vi "FlywheelVariableAngleControl.vi"(10 "Flywheel Commands":T1, 11 "Inputs_FlyWheel":T2={"Speed"=0.0, "Target Distance"=142.3980439543401}) -> (3 "Outputs_Flywheel":T3={"Wheel Speed"=9001.0})   [LabVIEW 2012]
uses:
  Outputs_Flywheel.ctl
  Sensor_Inputs_FlyWheel.ctl
  Input_Commands_Flywheel.ctl
panel:
  in  "Key Speed":dbl=2550.0
  in  "Reverse Speed":dbl=-400.0
  in  "Reset Speed":dbl=1300.0
  in  "Layup Speed":dbl=1300.0
  out "D out":dbl
  out "I out":dbl=0.003692626953125
  out "P out":dbl=0.399993896484375
  in  "Get PID":bool
  out "error out 2":errorcluster
  out "error out":errorcluster
  out "Average Speed":dbl
  in  "D":dbl
  in  "I":dbl=0.0037
  in  "P":dbl=0.6
  in  "SetPID":bool
  in  "Wheel Speed":dbl
  out "Current Speed":dbl(graph)
  # "Inputs"
  # "Constants"
  # "Outputs"
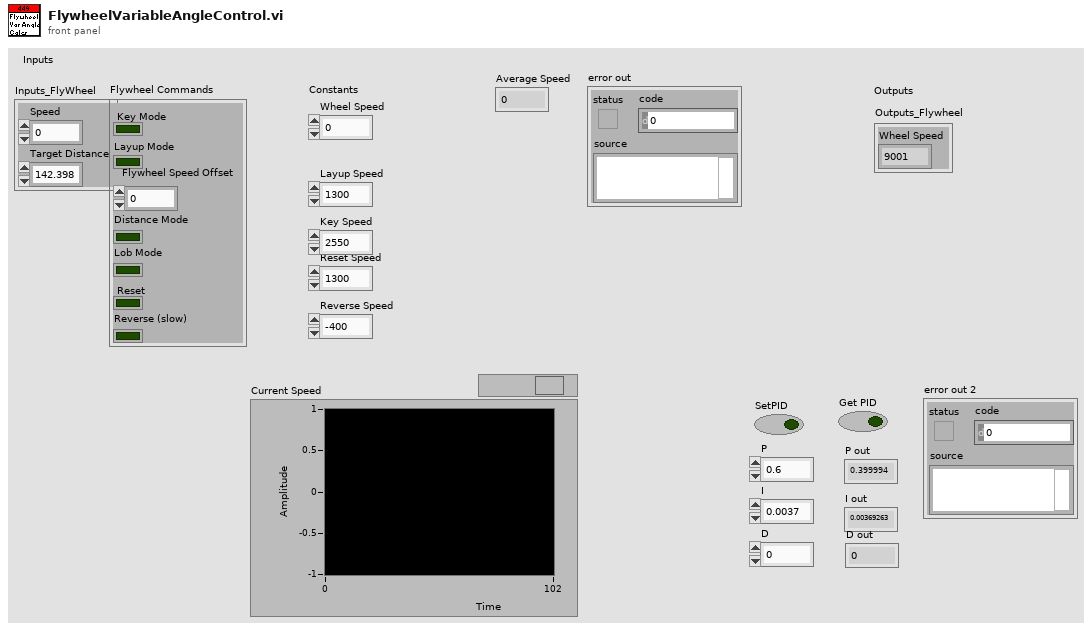
[diagram p1: front panel]
types:
  T1 = typedef "Input_Commands_Flywheel.ctl" = cluster{"Key Mode":bool, "Layup Mode":bool, "Flywheel Speed Offset":dbl, "Distance Mode":bool, "Lob Mode":bool, "Reset":bool, "Reverse (slow)":bool}
  T2 = typedef "Sensor_Inputs_FlyWheel.ctl" = cluster{"Speed":dbl, "Target Distance":dbl}
  T3 = typedef "Outputs_Flywheel.ctl" = cluster{"Wheel Speed":dbl}
  T4 = typedef "WPI_MotorControlDeviceRef.ctl" = cluster{"DeviceStatus":errorcluster, "Type":enum16{"PWM", "CAN"}, "PWM":cluster{"Digital Module":T5, "PWM Channel":T6, "DeadBand":T7}, "CAN":cluster{"Device Number":u8, "Control Mode":T8, "Semaphore":T9, "Max Vout":dbl}, "Invert":bool, "TransformRef":T10, "InvTransformRef":T10}
  T5 = typedef "FPGA_TypedefDigitalModule.ctl" = enum16{"Digital Module 1", "Digital Module 2"}
  T6 = typedef "FPGA_DIOPWMChannel.ctl" = enum8{"PWM 1", "PWM 2", "PWM 3", "PWM 4", "PWM 5", "PWM 6", "PWM 7", "PWM 8", "PWM 9", "PWM 10", "Invalid"}
  T7 = typedef "WPI_PWMDeadband.ctl" = cluster{"Name":string, "maxPositivePwm":i32, "minPositivePwm":i32, "centerPwm":i32, "maxNegativePwm":i32, "minNegativePwm":i32, "angularRange":u16}
  T8 = typedef "WPI_CANJaguar_ControlMode.ctl" = enum8{"Percent VBus", "Current", "Speed", "Position", "Voltage"}
  T9 = typedef "Semaphore RefNum" = refnum<k1>
  T10 = typedef "WPI_PWMTransform_ConPane.ctl" = refnum<vi>
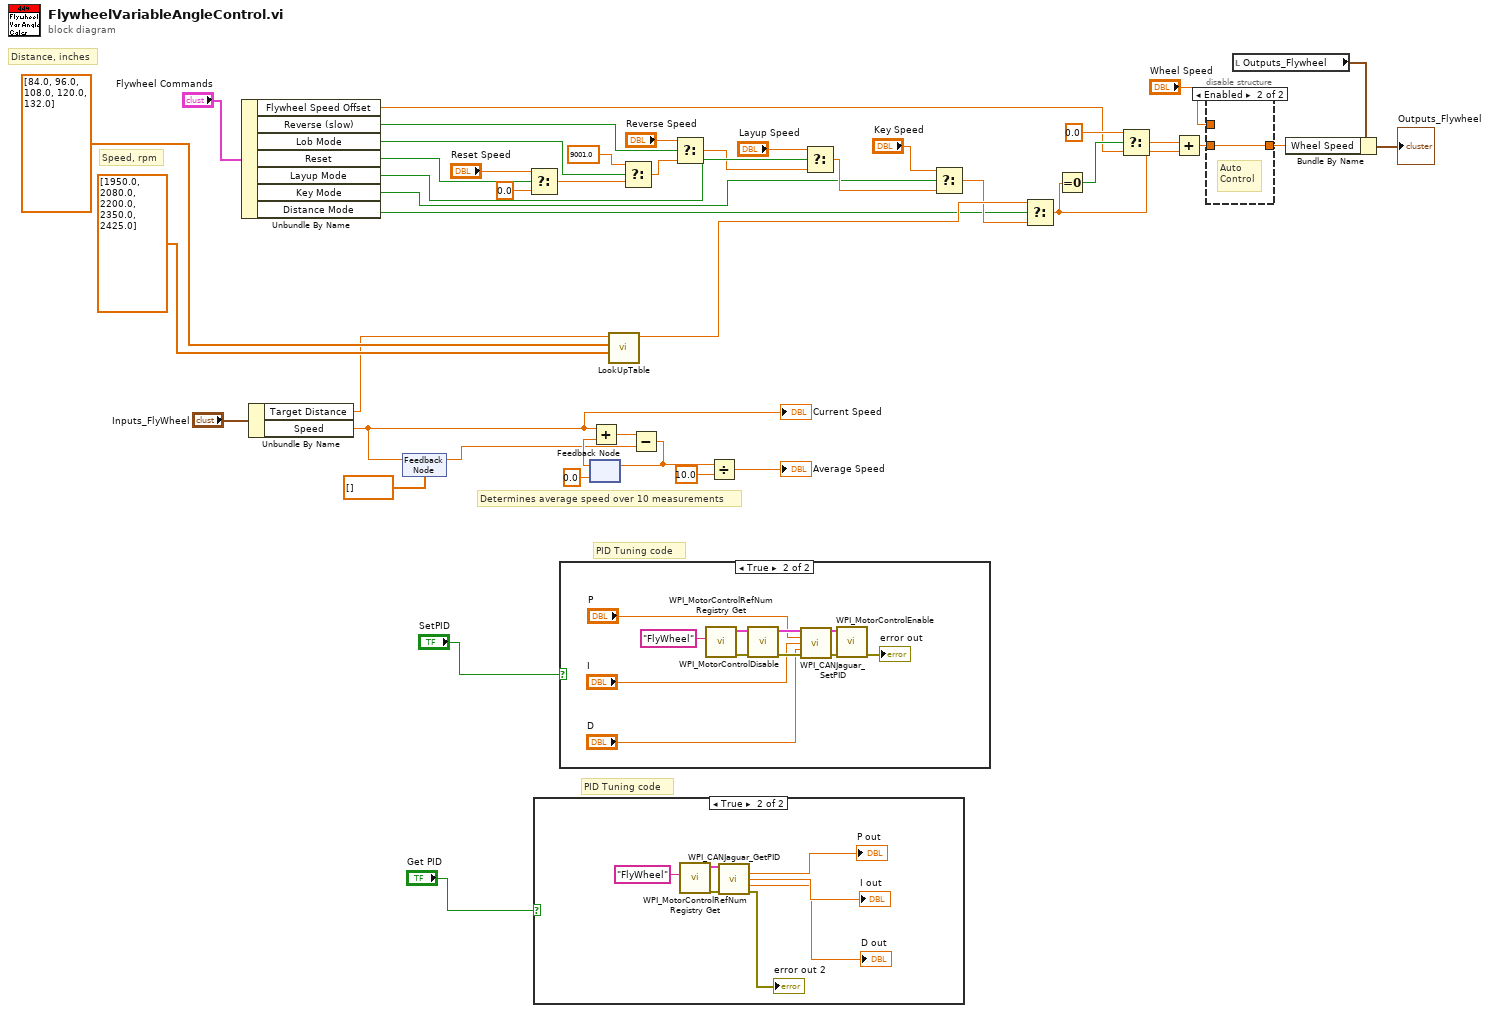
[diagram p0: block diagram]
diagram:
  # "Speed, rpm"
  # "Distance, inches"
  # "PID Tuning code"
  # "Determines average speed over 10 measurements"
  # "PID Tuning code"
  n1 = Unbundle By Name("Flywheel Commands") -> ("Flywheel Speed Offset"=w15:dbl, "Reverse (slow)"=w24:bool, "Lob Mode"=w27:bool, "Reset"=w2:bool, "Layup Mode"=w20:bool, "Key Mode"=w10:bool, "Distance Mode"=w7:bool)
  n2 = Unbundle By Name("Inputs_FlyWheel") -> ("Target Distance"=w6:dbl, "Speed"=w28:dbl)
  "Current Speed" <- w28
  n3 = feedback-in #1(w28) -> ()
  n4 = feedback #1(dbl[] []) -> (w38:dbl)
  n5 = Select(t="Reset Speed", s=w2, f=0.0) -> (s? t:f=w3:dbl)
  n6 = case shown="True" "Get PID" {
    frame False {
    }
    frame True {
      n7 = call <vilib>:"WPI_MotorControlRefNum Registry Get.vi"("refnum name"="FlyWheel") -> ("error out"=w49:errorcluster, "MotorControlDevRef"=w50:T4)  [unwired: 9 in]
      n8 = call <vilib>:"WPI_CANJaguar_GetPID.vi"("CAN Jaguar Ref"=w50, "error in (no error)"=w49) -> ("P"=→"P out":dbl, "I"=→"I out":dbl, "D"=→"D out":dbl, "error out"=→"error out 2":errorcluster)  [unwired: 9 in, 1 out]
    }
  }
  n9 = case shown="True" "SetPID" {
    frame False {
    }
    frame True {
      n10 = call <vilib>:"WPI_MotorControlRefNum Registry Get.vi"("refnum name"="FlyWheel") -> ("error out"=w61:errorcluster, "MotorControlDevRef"=w60:T4)  [unwired: 9 in]
      n11 = call <vilib>:"WPI_MotorControlDisable.vi"("error in (no error)"=w61, "MotorControlDevRef"=w60) -> ("error out"=w58:errorcluster, "MotorControlDevRef"=w59:T4)  [unwired: 8 in]
      n12 = call <vilib>:"WPI_CANJaguar_SetPID.vi"("CAN Jaguar Ref"=w59, "P"="P", "I"="I", "D"="D", "error in (no error)"=w58) -> ("CAN Jaguar Ref Out"=w57:T4, "error out"=w56:errorcluster)  [unwired: 9 in]
      n13 = call <vilib>:"WPI_MotorControlEnable.vi"("error in (no error)"=w56, "CAN Jaguar Ref"=w57) -> ("error out"=→"error out":errorcluster)  [unwired: 8 in, 1 out]
    }
  }
  n14 = feedback #2(0.0) -> (w40:dbl)
  n15 = Add(x=w28, y=w40) -> (x+y=w39:dbl)
  n16 = call "LookUpTable.vi"("Speeds"=dbl[] [1950.0, 2080.0, 2200.0, 2350.0, 2425.0], "Distances"=dbl[] [84.0, 96.0, 108.0, 120.0, 132.0], "Required Distance"=w6) -> ("Required Speed"=w9:dbl)  [unwired: 7 in, 1 out]
  n17 = Select(t=9001.0, s=w27, f=w3) -> (s? t:f=w25:dbl)
  n18 = Subtract(x=w39, y=w38) -> (x-y=w36:dbl)
  n19 = feedback-in #2(w36) -> ()
  n20 = Select(t="Reverse Speed", s=w24, f=w25) -> (s? t:f=w18:dbl)
  n21 = Divide(x=w36, y=10.0) -> (x/y=→"Average Speed":dbl)
  n22 = Select(t="Layup Speed", s=w20, f=w18) -> (s? t:f=w12:dbl)
  n23 = Select(t="Key Speed", s=w10, f=w12) -> (s? t:f=w8:dbl)
  n24 = Select(t=w9, s=w7, f=w8) -> (s? t:f=w5:dbl)
  n25 = Equal To 0?(x=w5) -> (x = 0?=w17:bool)
  n26 = Select(t=0.0, s=w17, f=w15) -> (s? t:f=w14:dbl)
  n27 = Add(x=w14, y=w5) -> (x+y=w13:dbl)
  n28 = disable-structure shown="Enabled" {
    disable-tunnel: [w63 w64] -> w33
    disable-tunnel: w13 -> [_ w64]
    disable-tunnel: "Wheel Speed" -> [w63 _]
    frame Disabled {
      # "Front\nPanel\nControl"
    }
    frame Enabled {
      # "Auto\nControl"
    }
  }
  n29 = local read "Outputs_Flywheel"() -> (w43:T3)
  n30 = Bundle By Name(cluster=w43, "Wheel Speed"=w33) -> (→"Outputs_Flywheel":T3)
